vi "Main RT.vi"() -> ()   [LabVIEW 2021]
uses:
  IP addresses.lvlib
panel:
  out "IPs availables":i32
  out "IP/Domain":string[](array[string])
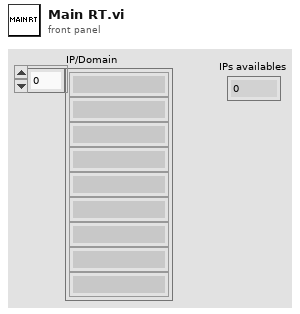
[diagram p1: front panel]
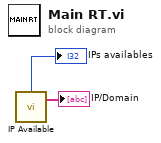
[diagram p0: block diagram]
diagram:
  n1 = call "IP Available.vi"() -> ("IPs availables"=→"IPs availables":i32, "IP/Domain"=→"IP/Domain":string[])  [unwired: 4 in]
